vi "Gespeicherte Werte.vi"(5 "Port changed in":bool, 6 "Aktionen":T3, 8 "AKTIV?":bool[](array[boolean]), 9 "Diverse Werte":T4={"Kalibriergaseingang"=0, "SamplePoint"=0, "CalGas zu PNS"=0, "Gas-Reihenfolge"=[], "Zeit 0-Gas"=0.0, "Zeit CalGas"=0.0, "AK Befehlssatz"=enum."IAG v1.4"}, 10 "TCP Parameter":T1={"Port"=3615, "Timeout"=30}, 11 "Serielle Parameter":T2={"VISA resource name"="COM1", "baud rate"=38400, "data bits"=8, "parity"=0, "stop bits"=10, "flow control"=0} {"flow control" items=["None"=0, "XON/XOFF"=1, "RTS/CTS"=2, "DTR/DSR"=4]; "stop bits" items=["1.0"=10, "1.5"=15, "2.0"=20]; "parity" items=["None", "Odd", "Even", "Mark", "Space"]; "data bits" min=5 max=8 step=1}) -> (0 "AKTIV?":bool[](array[boolean]), 1 "Diverse Werte":T4={"Kalibriergaseingang"=0, "SamplePoint"=0, "CalGas zu PNS"=0, "Gas-Reihenfolge"=[], "Zeit 0-Gas"=0.0, "Zeit CalGas"=0.0, "AK Befehlssatz"=enum."IAG v1.4"}, 2 "TCP Parameter":T1={"Port"=3615, "Timeout"=30}, 3 "Serielle Parameter":T2={"VISA resource name"="COM1", "baud rate"=38400, "data bits"=8, "parity"=0, "stop bits"=10, "flow control"=0} {"flow control" items=["None"=0, "XON/XOFF"=1, "RTS/CTS"=2, "DTR/DSR"=4]; "stop bits" items=["1.0"=10, "1.5"=15, "2.0"=20]; "parity" items=["None", "Odd", "Even", "Mark", "Space"]; "data bits" min=5 max=8 step=1}, 4 "Port changed out":bool)   [LabVIEW 2020, in "AK-Schnittstelle.lvlib"]
uses:
  AK-Schnittstelle.lvlib
  Diverse gespeicherte Werte.ctl
  AK Befehlssatz.ctl
  Aktionen Gespeicherte Werte.ctl
  Serielle Parameter.ctl
  AK TCP/TCP Parameter.ctl
  Visualisierungs Elemente/String - Ausgabefeld.ctl
  SysLog/SysLog Interface.ctl
  Allgemein/allgemeine Sub-VIs.lvlib
  SysLog/SysLog.lvlib
  <vilib>/Utility/Data Type/NI_Data Type.lvlib
  AK Seriell/AK Seriell.lvlib
  AK TCP/AK TCP.lvlib
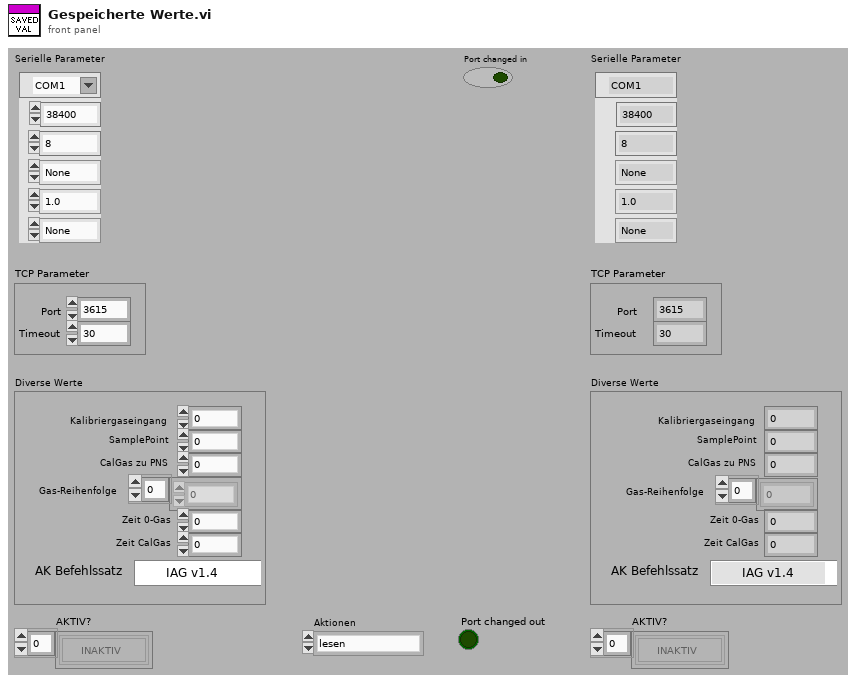
[diagram p1: front panel]
types:
  T1 = typedef "AK-Schnittstelle.lvlib/AK TCP.lvlib/TCP Parameter.ctl" = cluster{"Port":u16, "Timeout":u16}
  T2 = typedef "AK-Schnittstelle.lvlib/AK Seriell.lvlib/Serielle Parameter.ctl" = cluster{"VISA resource name":refnum<visa-resource-name>, "baud rate":u32, "data bits":u16, "parity":u16, "stop bits":u16, "flow control":u16}
  T3 = typedef "AK-Schnittstelle.lvlib/Aktionen Gespeicherte Werte.ctl" = enum16{"lesen", "laden", "speichern", "Seriell", "TCP", "Diverse", "AKTIV", "AK-Namen"}
  T4 = typedef "AK-Schnittstelle.lvlib/Diverse gespeicherte Werte.ctl" = cluster{"Kalibriergaseingang":i16, "SamplePoint":i16, "CalGas zu PNS":i16, "Gas-Reihenfolge":i16[], "Zeit 0-Gas":sgl, "Zeit CalGas":sgl, "AK Befehlssatz":T5}
  T5 = typedef "AK-Schnittstelle.lvlib/AK Befehlssatz.ctl" = enum16{"MEXA", "IAG v1.4", "AVL (Puma)", "PEUS"}
  T6 = typedef "String - Ausgabefeld.ctl" = string
  T7 = typedef "SysLog.lvlib/SysLog Interface.ctl" = cluster{"FehlermeldungsCode":i32, "ErfolgsmeldungsCode":i32, "ParameterListenString":string, "Anzeige":bool, "SysLogIcon":enum16{"OK", "Warnung", "Fehler"}, "intern":bool}
  T8 = cluster{"Serielle Parameter":T2, "TCP Parameter":T1, "Diverse Werte":T4, "AKTIV?":bool[], "AK Namen":T6[]}
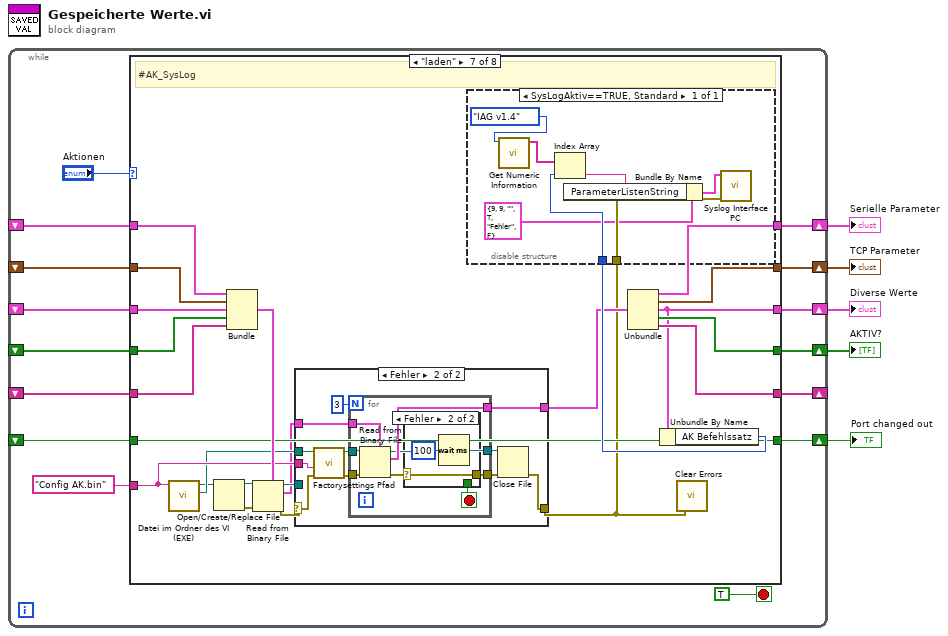
[diagram p0: block diagram]
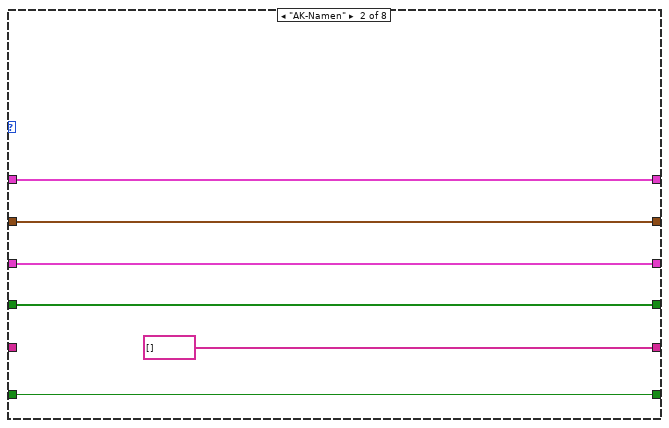
[diagram p3: hidden frame]
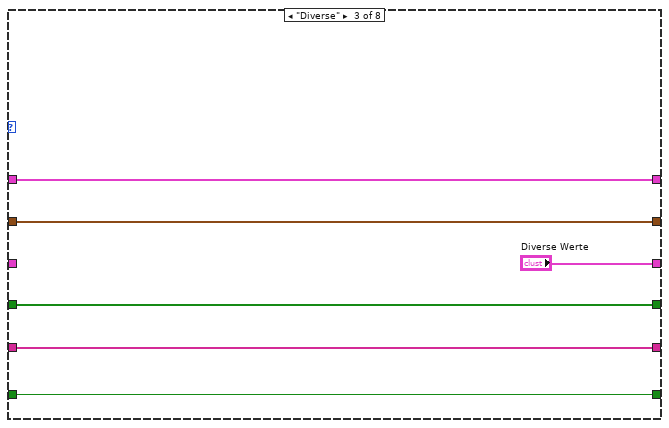
[diagram p4: hidden frame]
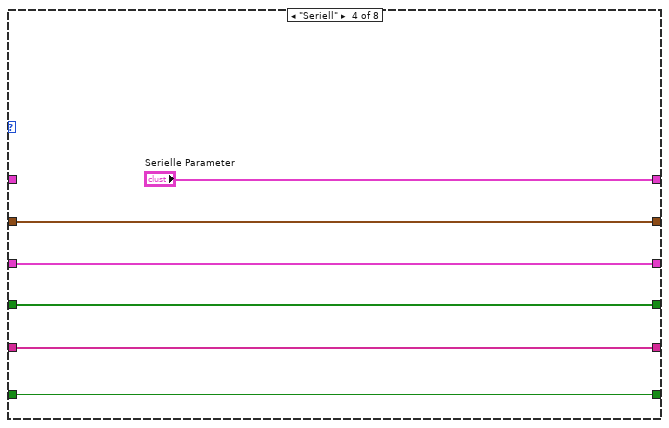
[diagram p5: hidden frame]
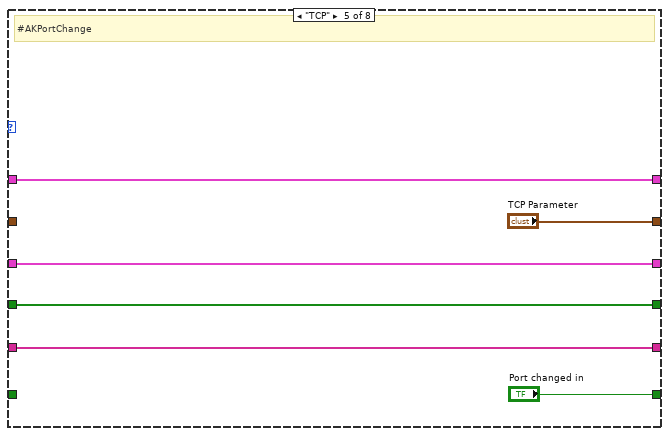
[diagram p6: hidden frame]
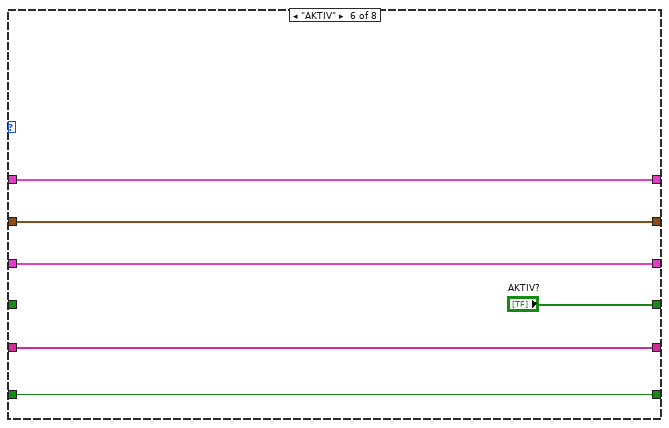
[diagram p7: hidden frame]
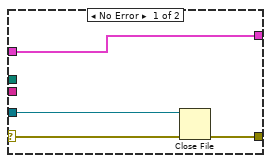
[diagram p8: hidden frame]
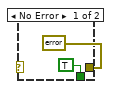
[diagram p9: hidden frame]
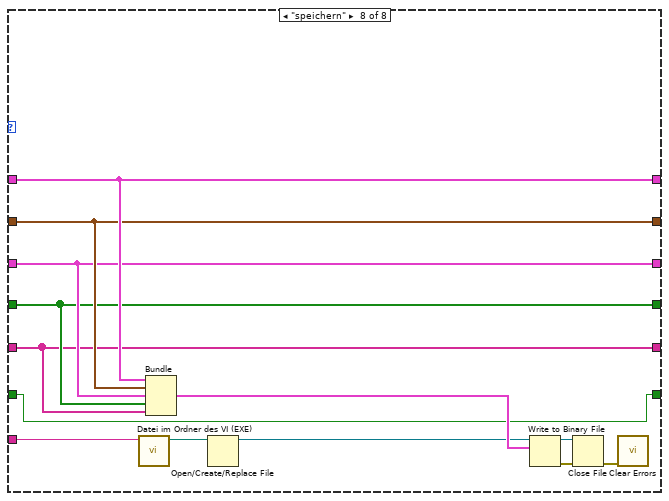
[diagram p10: hidden frame]
diagram:
  n1 = while {
    shift-right: [w19] -> w5
    shift-left: _ -> [w17]
    shift-right: [w12] -> w4
    shift-left: _ -> [w13]
    shift-right: [w15] -> w3
    shift-left: _ -> [w14]
    shift-right: [w10] -> w2
    shift-left: _ -> [w11]
    shift-right: [w8] -> _
    shift-left: _ -> [w9]
    shift-right: [w7] -> w1
    shift-left: _ -> [w6]
    stop <- TRUE stop-if-true
    n2 = case shown="\"laden\"" "Aktionen" {
      tunnel: [w26 w32 "Diverse Werte" w43 w49 w54 w69 w123] -> w19
      tunnel: w17 -> [w26 w32 _ w43 w49 w54 w77 w123]
      tunnel: "Config AK.bin" ("Dateiname") -> [_ _ _ _ _ _ w65 w126]
      tunnel: [w25 w31 w37 "Serielle Parameter" w48 w56 w75 w125] -> w15
      tunnel: w14 -> [w25 w31 w37 _ w48 w56 w79 w125]
      tunnel: w13 -> [w24 w30 w36 w42 _ w55 w78 w124]
      tunnel: [w24 w30 w36 w42 "TCP Parameter" w55 w74 w124] -> w12
      tunnel: w11 -> [w23 w29 w35 w41 w47 _ w72 w122]
      tunnel: [w23 w29 w35 w41 w47 "AKTIV?" w73 w122] -> w10
      tunnel: w9 -> [w22 _ w34 w40 w46 w52 w71 w121]
      tunnel: [w22 T6[] [] ("AK Namen") w34 w40 w46 w52 w70 w121] -> w8
      tunnel: [w21 w27 w33 w39 "Port changed in" w51 w67 w119] -> w7
      tunnel: w6 -> [w21 w27 w33 w39 _ w51 w67 w119]
      frame "lesen", Default {
      }
      frame "AK-Namen" {
      }
      frame "Diverse" {
      }
      frame "Seriell" {
      }
      frame "TCP" {
        # "#AKPortChange"
      }
      frame "AKTIV" {
      }
      frame "laden" {
        # "#AK_SysLog"
        n3 = call "Datei im Ordner des VI (EXE).vi"("Dateiname"=w65) -> ("Ordner des Haupt-VIs"=w63:path, "Dateipfad im Ordner des Haupt-VIs"=w57:path)  [unwired: 8 in, 1 out]
        n4 = Open/Create/Replace File(file path (use dialog)=w57) -> (refnum out=w58:refnum<file>, error out=w59:errorcluster)  [unwired: 5 in, 1 out]
        n5 = Bundle("Serielle Parameter"=w79, "TCP Parameter"=w78, "Diverse Werte"=w77, "AKTIV?"=w72, "AK Namen"=w71) -> (w76:T8)  [unwired: 1 in]
        n6 = Read from Binary File(5:w76, 8:w59, 11:w58) -> (0:w66:errorcluster, 2:w62:T8, 3:w64:refnum<file>)  [unwired: 4 out]
        n7 = case shown="Fehler" w66 {
          selector: w66 -> [w82 w86]
          tunnel: w63 -> [_ w87]
          tunnel: w62 -> [w83 w85]
          tunnel: [w83 w93] -> w61
          tunnel: [w80 w91] -> w60
          tunnel: w64 -> [w81 _]
          tunnel: w65 -> [_ w84]
          frame No Error {
            n8 = Close File(refnum=w81, error in=w82) -> (error out=w80:errorcluster)  [unwired: 1 out]
          }
          frame Error {
            n9 = call "Factorysettings Pfad.vi"("error in (no error)"=w86, "Dateiname"=w84, "Ordner des Haupt-VIs"=w87) -> ("error out"=w88:errorcluster, "Pfad Factorysettings"=w89:path)  [unwired: 7 in]
            n10 = for {
              N: 3 -> [_]
              tunnel: w88 -> [w100]
              tunnel: w89 -> [w99]
              tunnel: [w98] -> w93
              tunnel: [w97] -> w92
              tunnel: [w96] -> w90
              tunnel: w85 -> [w95]
              stop <- w101 stop-if-true
              n11 = Read from Binary File(5:w95, 8:w100, 11:w99) -> (0:w102:errorcluster, 2:w98:T8, 3:w96:refnum<file>)  [unwired: 3 in, 1 out]
              n12 = case shown="Fehler" w102 {
                selector: w102 -> [_ w105]
                tunnel: [TRUE _] -> w101
                tunnel: [errorcluster {"status"=FALSE, "code"=0, "source"=""} ("error IO") w105] -> w97
                frame No Error {
                }
                frame Error {
                  n13 = Wait (ms)(milliseconds to wait=u32 100 ("Zu wartende ms")) -> ()  [unwired: 1 out]
                }
              }
            }
            n14 = Close File(refnum=w90, error in=w92) -> (error out=w91:errorcluster)  [unwired: 1 out]
          }
        }
        n15 = Unbundle(w61) -> ("Serielle Parameter"=w75:T2, "TCP Parameter"=w74:T1, "Diverse Werte"=w69:T4, "AKTIV?"=w73:bool[], "AK Namen"=w70:T6[])
        n16 = Unbundle By Name(w69) -> ("AK Befehlssatz"=w68:T5)
        n17 = disable-structure shown="SysLogAktiv==TRUE, Standard" {
          disable-tunnel: w68 -> [w111]
          disable-tunnel: w60 -> [w110]
          frame condition #0 (active) {
            n18 = call <vilib>:"Get Numeric Information.vi"("variant"=AK_Befehlssatz."IAG v1.4" ("AK Befehlssatz")) -> ("enum names"=w112:string[])  [unwired: 7 in, 3 out]
            n19 = Index Array(array=w112, index=w111) -> (element=w108:string)
            n20 = Bundle By Name(cluster=T7 {"FehlermeldungsCode"=9, "ErfolgsmeldungsCode"=9, "ParameterListenString"="", "Anzeige"=TRUE, "SysLogIcon"=enum."Fehler", "intern"=FALSE} ("Cluster (in)"), "ParameterListenString"=w108) -> (w107:T7)
            n21 = call "Syslog Interface PC.vi"("Fehler (in)"=w110, "Cluster (in)"=w107) -> ()  [unwired: 9 in, 1 out]
          }
        }
        n22 = call <vilib>:"Clear Errors.vi"("error in (no error)"=w60) -> ()  [unwired: 5 in, 2 out]
      }
      frame "speichern" {
        n23 = call "Datei im Ordner des VI (EXE).vi"("Dateiname"=w126) -> ("Dateipfad im Ordner des Haupt-VIs"=w118:path)  [unwired: 8 in, 2 out]
        n24 = Bundle("Serielle Parameter"=w125, "TCP Parameter"=w124, "Diverse Werte"=w123, "AKTIV?"=w122, "AK Namen"=w121) -> (w120:T8)  [unwired: 1 in]
        n25 = Open/Create/Replace File(file path (use dialog)=w118) -> (refnum out=w117:refnum<file>)  [unwired: 5 in, 2 out]
        n26 = Write to Binary File(file (use dialog)=w117, data=w120) -> (refnum out=w114:refnum<file>, error out=w115:errorcluster)  [unwired: 1 in, 4 out]
        n27 = Close File(refnum=w114, error in=w115) -> (error out=w116:errorcluster)  [unwired: 1 out]
        n28 = call <vilib>:"Clear Errors.vi"("error in (no error)"=w116) -> ()  [unwired: 5 in, 2 out]
      }
    }
  }
  "Diverse Werte" <- w5
  "Serielle Parameter" <- w3
  "TCP Parameter" <- w4
  "AKTIV?" <- w2
  "Port changed out" <- w1
